vi "stop software.vi"() -> ()   [LabVIEW 2020]
panel:
  in  "stop software":bool
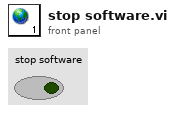
[diagram p1: front panel]
diagram:
